vi "pattern sub.vi"() -> ()   [LabVIEW 2020]
panel:
  out "String 3":string
  out "concatenated string":string
  out "String 2":string
  out "String":string
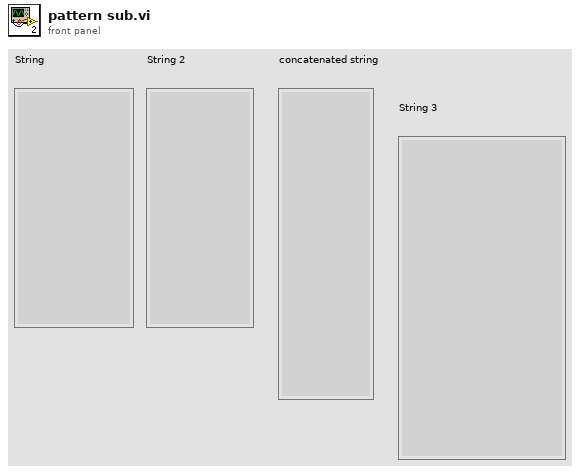
[diagram p1: front panel]
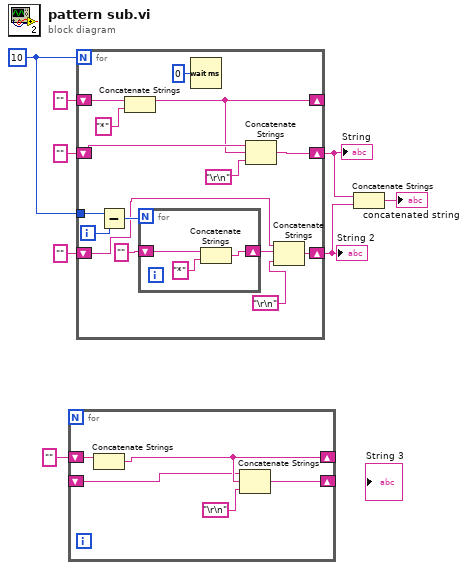
[diagram p0: block diagram]
diagram:
  w8 = 10
  n1 = for {
    shift-right: [w11] -> _
    shift-left: "" -> [w13]
    shift-right: [w12] -> _
    shift-left: _ -> [w10]
    n2 = Concatenate Strings(w13) -> (w11:string)  [unwired: 1 in]
    n3 = Concatenate Strings(w10, w11, "\r\n") -> (w12:string)
  }
  n4 = for {
    N: w8 -> [_]
    shift-right: [w23] -> _
    shift-left: "" -> [w27]
    shift-right: [w26] -> w4
    shift-left: "" -> [w24]
    tunnel: w8 -> [w21]
    shift-right: [w16] -> w3
    shift-left: "" -> [w15]
    i -> [w20]
    n5 = Subtract(x=w21, y=w20) -> (x-y=w19:i32)
    n6 = Concatenate Strings(w27, "*" ("string")) -> (w23:string)
    n7 = for {
      N: w19 -> [_]
      shift-right: [w29] -> w17
      shift-left: "" -> [w30]
      n8 = Concatenate Strings(w30, "*" ("string")) -> (w29:string)
    }
    n9 = Wait (ms)(milliseconds to wait=u32 0 ("millisecond timer value")) -> ()  [unwired: 1 out]
    n10 = Concatenate Strings(w24, w23, "\r\n") -> (w26:string)
    n11 = Concatenate Strings(w15, w17, "\r\n") -> (w16:string)
  }
  "String" <- w4
  "String 2" <- w3
  n12 = Concatenate Strings(w4, w3) -> (→"concatenated string":string)
